vi "Read StrArrayList.vi"(8 "error in (no error)":errorcluster, 11 "OOPbyRef in":refnum<class "OOPbyRef.lvclass">) -> (0 "error out":errorcluster, 3 "OOPbyRef out":refnum<class "OOPbyRef.lvclass">)   [LabVIEW 2021, in "DQMH_byOOPRef.lvlib" / "OOPbyRef.lvclass"]
uses:
  OOPbyRef.lvclass
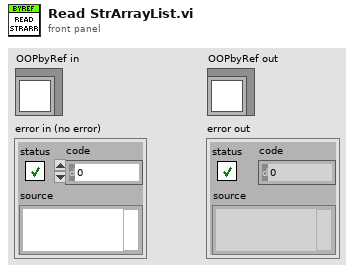
[diagram p1: front panel]
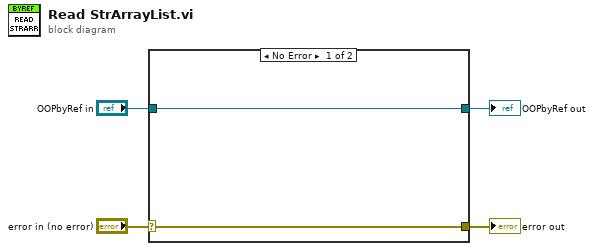
[diagram p0: block diagram]
diagram:
  n1 = case shown="No Error" "error in (no error)" {
    selector: "error in (no error)" -> [w5 w8]
    tunnel: [w5 w8] -> w3
    tunnel: [w6 w7] -> w1
    tunnel: "OOPbyRef in" -> [w6 w7]
    frame No Error {
    }
    frame Error {
    }
  }
  "error out" <- w3
  "OOPbyRef out" <- w1
